vi "Layer Scan V4.vi"() -> ()   [LabVIEW 2024]
uses:
  <vilib>/DAQmx/write.llb/DAQmx Write (Analog 1D DBL NChan 1Samp).vi
  <vilib>/DAQmx/create/channels.llb/DAQmx Create Channel (AO-Voltage-Basic).vi
  <vilib>/DAQmx/miscellaneous.llb/DAQmx Fill In Error Info.vi
  <instrlib>/niScope/Configure/Trigger/niScope Configure Trigger Software.vi
  <instrlib>/niScope/Acquire/Fetch/niScope Fetch Cluster.vi
panel:
  in  "Channel Name 2":string="0" caption="Channel(s)"
  in  "Resource Name 2":refnum<k15>="Dev1" caption="Resource Name(s)"
  in  "Min. Sample Rate 2":dbl=10000000.0 caption="Min. Sample Rate" format="%#_6p"
  in  "Vertical Range (V) 2":dbl=2.0 caption="Vertical Range (V)" format="%_3g"
  out "Waveform from Scope":T1(graph)
  in  "Max. Points per Fetch":i32=1000
  in  "Plot Data?":bool=TRUE
  out "Last Points Fetched":i32
  out "Total Points Fetched":i32
  in  "Simulate?":bool
  out "decimated array 2":dbl[](array[numeric])
  out "decimated array":dbl[](array[numeric])
  out "Y coord filename":i32
  out "x coord file name":i32
  out "Filename Out":path
  in  "Data File Name":path
  in  "Data folder Path":path
  in  "X offset":dbl
  in  "Y offset":dbl
  in  "distance":dbl
  in  "Y Count":dbl
  in  "X Count":dbl
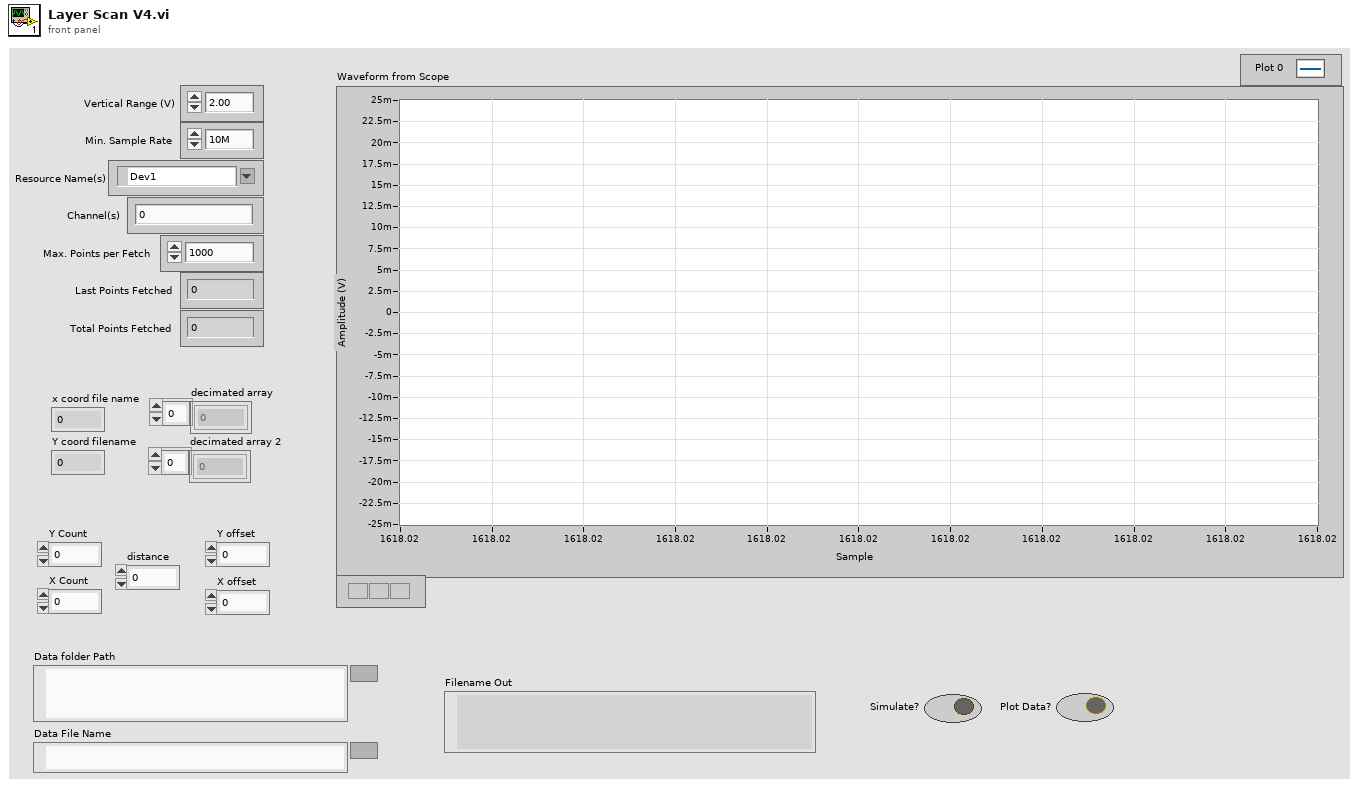
[diagram p1: front panel]
types:
  T1 = cluster{"relativeInitialX":dbl, "xIncrement":dbl, "wfm":dbl[]}
  T2 = cluster{"actualSamples":i32, "absoluteInitialX":dbl, "relativeInitialX":dbl, "xIncrement":dbl, "offset":dbl, "gain":dbl, "reserved1":dbl, "reserved2":dbl}
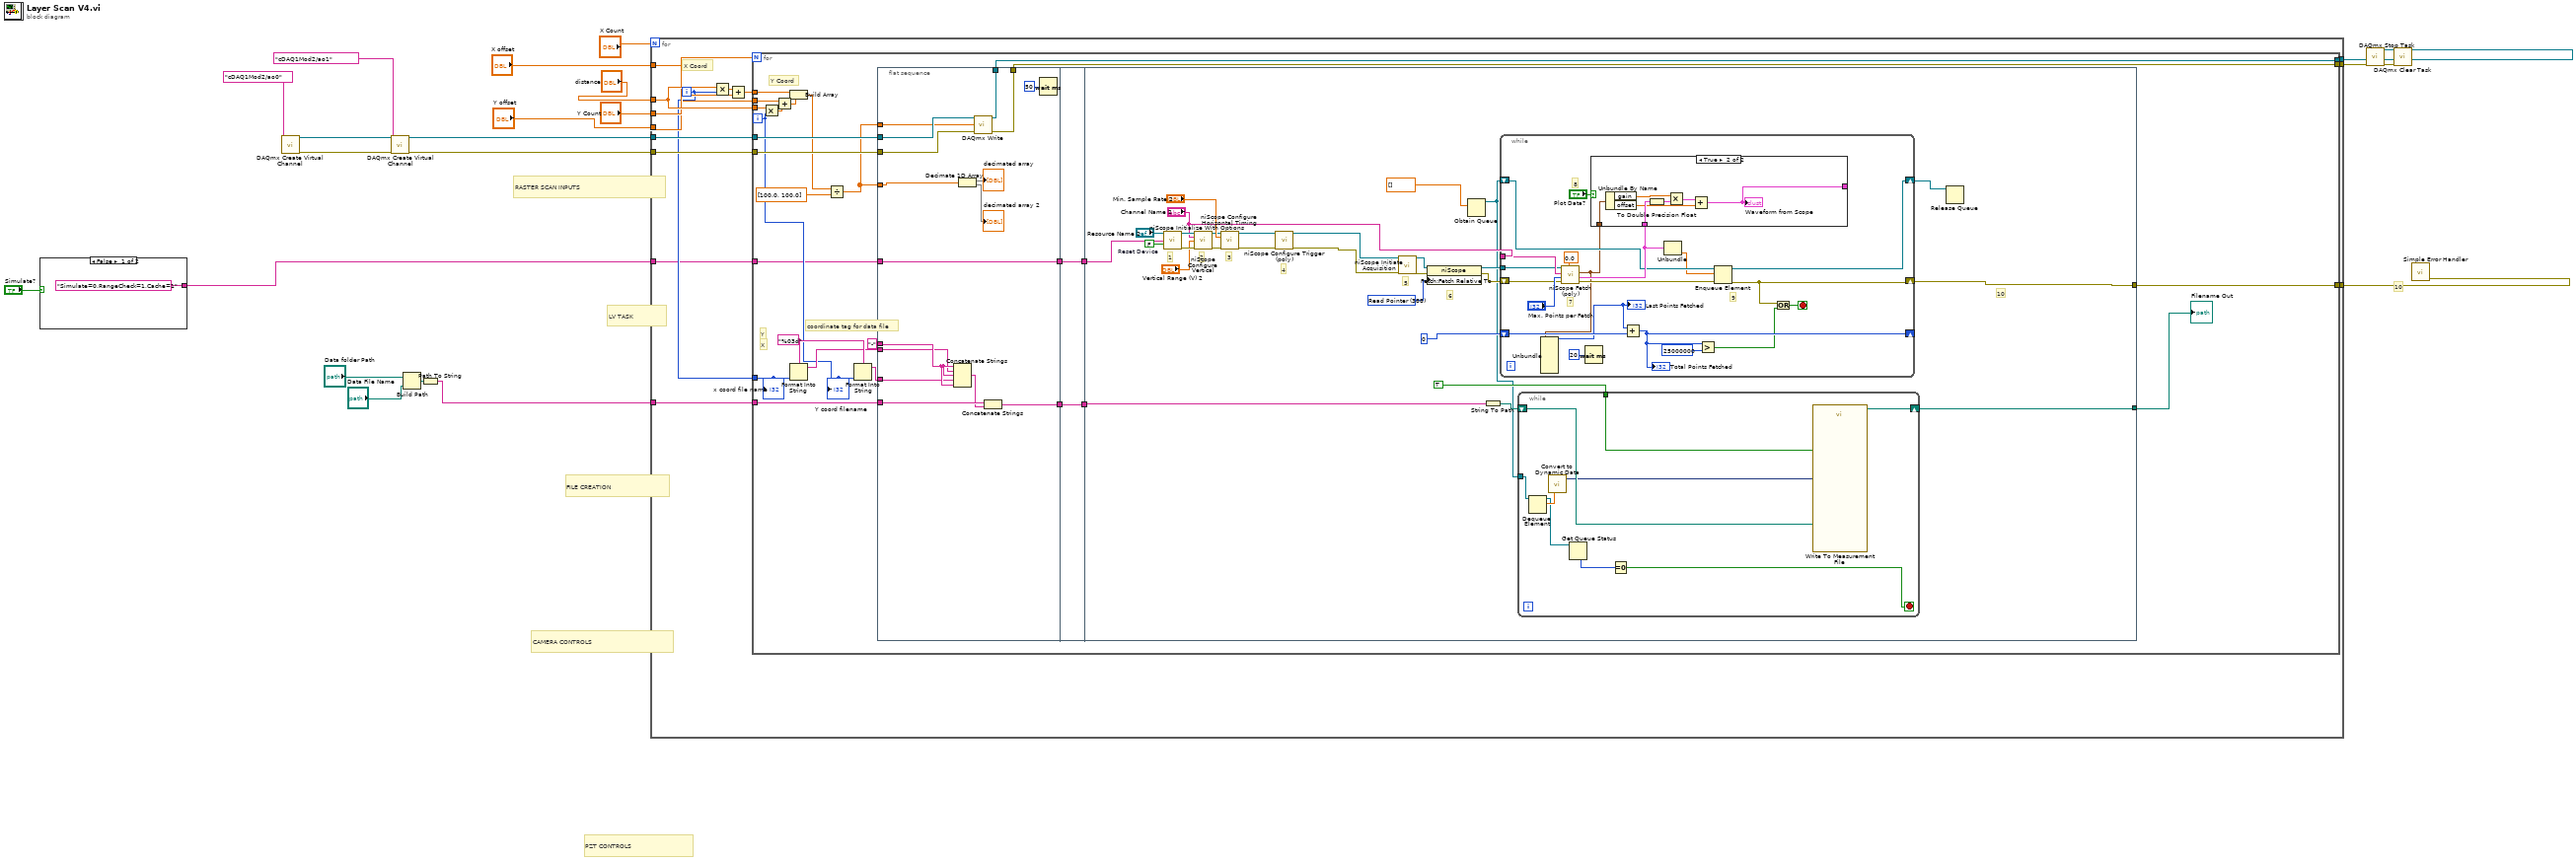
[diagram p0: block diagram]
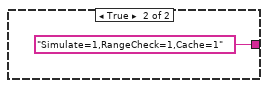
[diagram p2: hidden frame]
diagram:
  # "10"
  # "FILE CREATION"
  # "PZT CONTROLS"
  # "CAMERA CONTROLS"
  # "LV TASK"
  # "RASTER SCAN INPUTS"
  n1 = case shown="False" "Simulate?" {
    tunnel: ["Simulate=0,RangeCheck=1,Cache=1" ("option string") "Simulate=1,RangeCheck=1,Cache=1" ("option string")] -> w1
    frame False {
    }
    frame True {
    }
  }
  n2 = call-poly <vilib>:"DAQmx Create Virtual Channel.vi"("physical channels"=tag "cDAQ1Mod2/ao0") -> ("task out"=w15:refnum<k21>, "error out"=w14:errorcluster)  [unwired: 13 in]
  n3 = call-poly <vilib>:"DAQmx Create Virtual Channel.vi"("task in"=w15, "physical channels"=tag "cDAQ1Mod2/ao1", "error in"=w14) -> ("task out"=w13:refnum<k21>, "error out"=w12:errorcluster)  [unwired: 11 in]
  n4 = Build Path(base path="Data folder Path", name or relative path="Data File Name") -> (appended path=w5:path)
  n5 = Path To String(path=w5) -> (string=w4:string)
  n6 = for {
    N: "X Count" -> [_]
    tunnel: "distance" -> [w38]
    tunnel: "Y Count" -> [w37]
    tunnel: "Y offset" -> [w36]
    tunnel: "X offset" -> [w34]
    tunnel: w13 -> [w32]
    tunnel: w12 -> [w31]
    tunnel: [w30] -> w11
    tunnel: [w29] -> w10
    tunnel: [w28] -> w2
    tunnel: w4 -> [w27]
    tunnel: w1 -> [w25]
    i -> [w26]
    # "X Coord"
    n7 = Multiply(x=w38, y=w26) -> (x*y=w35:dbl)
    n8 = Add(x=w35, y=w34) -> (x+y=w33:dbl)
    n9 = for {
      N: w37 -> [_]
      tunnel: w38 -> [w64]
      tunnel: w36 -> [w62]
      tunnel: w33 -> [w61]
      tunnel: w32 -> [w59]
      tunnel: w31 -> [w58]
      tunnel: [w56] -> w30
      tunnel: [w55] -> w29
      tunnel: [w43] -> w28
      tunnel: w27 -> [w50]
      tunnel: w26 -> [w46]
      tunnel: w25 -> [w39]
      i -> [w45]
      w54 = "%03d" ("format string")
      # "coordinate tag for data file"
      # "X"
      # "Y"
      # "Y Coord"
      n10 = Multiply(x=w64, y=w45) -> (x*y=w63:dbl)
      n11 = Add(x=w62, y=w63) -> (x+y=w60:dbl)
      n12 = Format Into String(format string=w54, w46) -> (resulting string=w52:string)  [unwired: 2 in, 1 out]
      n13 = Build Array(w61, w60) -> (w57:dbl[])
      n14 = Divide(x=w57, y=dbl[] [100.0, 100.0]) -> (x/y=w44:dbl[])
      n15 = Format Into String(format string=w54, w45) -> (resulting string=w51:string)  [unwired: 2 in, 1 out]
      n16 = flat-sequence {
        tunnel: w59 -> [w79]
        tunnel: w58 -> [w78]
        tunnel: [w77] -> w56
        tunnel: [w76] -> w55
        tunnel: "-" ("string") -> [w75]
        tunnel: w52 -> [w74]
        tunnel: w51 -> [w73]
        tunnel: w50 -> [w72]
        tunnel: [w70] -> w49
        tunnel: w44 -> [w69]
        tunnel: w44 -> [w68]
        tunnel: [w65] -> w41
        tunnel: w39 -> [w65]
        tunnel: w49 -> [w82]
        tunnel: [w82] -> w48
        tunnel: w41 -> [w81]
        tunnel: [w81] -> w40
        tunnel: w48 -> [w110]
        tunnel: [w83] -> w43
        tunnel: [w87] -> w42
        tunnel: w40 -> [w90]
        frame #0 {
          n17 = Concatenate Strings(w75, w74, w75, w73, w75) -> (w71:string)
          n18 = Decimate 1D Array(w68) -> (→"decimated array":dbl[], →"decimated array 2":dbl[])
          n19 = call-poly <vilib>:"DAQmx Write.vi"("task/channels in"=w79, "data"=w69, "error in"=w78) -> ("task out"=w77:refnum<k21>, "error out"=w76:errorcluster)  [unwired: 10 in, 1 out]
          n20 = Concatenate Strings(w72, w71) -> (w70:string)
          n21 = Wait (ms)(milliseconds to wait=u32 50) -> ()  [unwired: 1 out]
        }
        frame #1 {
        }
        frame #2 {
          w101 = FALSE  # Reset Device
          w106 = 388 items=["Start"=482, "Trigger"=483, "Pretrigger"=477, "Now"=481, "Read Pointer"=388] ("Fetch:Fetch Relative To")
          # "4"
          # "3"
          # "2"
          # "1"
          # "10"
          # "6"
          # "5"
          n22 = call <instrlib>:"niScope Initialize With Options.vi"("resource name"="Resource Name 2", "option string"=w90, "reset device"=w101) -> ("instrument handle"=w103:refnum<k15>, "error out"=w102:errorcluster)  [unwired: 11 in]
          n23 = call <instrlib>:"niScope Configure Vertical.vi"("instrument handle"=w103, "channels"="Channel Name 2", "vertical range"="Vertical Range (V) 2", "error in"=w102) -> ("instrument handle out"=w95:refnum<k15>, "error out"=w94:errorcluster)  [unwired: 10 in]
          n24 = call <instrlib>:"niScope Configure Horizontal Timing.vi"("instrument handle"=w95, "min sample rate"="Min. Sample Rate 2", "error in"=w94) -> ("instrument handle out"=w99:refnum<k15>, "error out"=w100:errorcluster)  [unwired: 11 in]
          n25 = call-poly <instrlib>:"niScope Configure Trigger (poly).vi"("instrument handle"=w99, "error in"=w100) -> ("instrument handle out"=w92:refnum<k15>, "error out"=w91:errorcluster)  [unwired: 12 in]
          n26 = call <instrlib>:"niScope Initiate Acquisition.vi"("instrument handle"=w92, "error in"=w91) -> ("instrument handle out"=w107:refnum<k15>, "error out"=w108:errorcluster)  [unwired: 12 in]
          n27 = property class="niScope"(reference=w107, error in=w108, "Fetch:Fetch Relative To"=w106) -> (reference out=w104:refnum<k15>, error out=w105:errorcluster)
          n28 = Obtain Queue(element data type=dbl[] []) -> (queue out=w85:refnum<queue>)  [unwired: 4 in, 2 out]
          n29 = String To Path(string=w110) -> (path=w88:path)
          n30 = while {
            shift-left: 0 -> [w139]
            shift-right: [w130] -> _
            tunnel: "Channel Name 2" -> [w137]
            tunnel: w104 -> [w133]
            shift-right: [w126] -> w83
            shift-left: w105 -> [w132]
            shift-right: [w122] -> w86
            shift-left: w85 -> [w124]
            stop <- w138 stop-if-true
            # "9"
            # "8"
            # "7"
            n31 = call-poly <instrlib>:"niScope Fetch (poly).vi"("timeout"=0.0, "error in"=w132, "numSamples"="Max. Points per Fetch", "channels"=w137, "instrument handle"=w133) -> ("error out"=w127:errorcluster, "waveform"=w125:T1, "wfm info"=w121:T2)  [unwired: 3 in, 1 out]
            n32 = Unbundle(w121) -> ("actualSamples"=w120:i32)  [unwired: 7 out]
            "Last Points Fetched" <- w120
            n33 = Wait (ms)(milliseconds to wait=u32 20) -> ()  [unwired: 1 out]
            n34 = case shown="True" "Plot Data?" {
              tunnel: w125 -> [_ w145]
              tunnel: w121 -> [_ w146]
              tunnel: [_ w140] -> _
              frame False {
              }
              frame True {
                n35 = Unbundle By Name(w146) -> ("gain"=w144:dbl, "offset"=w142:dbl)
                n36 = To Double Precision Float(number=w145) -> (double precision float=w141:T1)
                n37 = Multiply(x=w144, y=w141) -> (x*y=w143:T1)
                n38 = Add(x=w143, y=w142) -> (x+y=w140:T1)
                "Waveform from Scope" <- w140
              }
            }
            n39 = Add(x=w120, y=w139) -> (x+y=w130:i32)
            "Total Points Fetched" <- w130
            n40 = Unbundle(w125) -> ("wfm"=w123:dbl[])  [unwired: 2 out]
            n41 = Greater?(x=w130, y=25000000) -> (0:w128:bool)
            n42 = Enqueue Element(queue=w124, element=w123, error in (no error)=w127) -> (queue out=w122:refnum<queue>, error out=w126:errorcluster)  [unwired: 1 in, 1 out]
            n43 = Or(x=w126, y=w128) -> (x .or. y?=w138:bool)
          }
          n44 = while {
            tunnel: TRUE ("Enable") -> [w119]
            tunnel: w85 -> [w115]
            shift-right: [w117] -> w87
            shift-left: w88 -> [w118]
            stop <- w111 stop-if-true
            n45 = Dequeue Element(queue=w115) -> (queue out=w113:refnum<queue>, element=w116:dbl[])  [unwired: 2 in, 2 out]
            n46 = call "Convert to Dynamic Data"("Array"=w116) -> ("Dynamic Data Type"=w114:dynamicdata)  [unwired: 3 in]
            n47 = Get Queue Status(queue=w113) -> (# elements in queue=w112:i32)  [unwired: 2 in, 7 out]
            n48 = Equal To 0?(x=w112) -> (x = 0?=w111:bool)
            n49 = call "Write To Measurement File"("Signals"=w114, "Enable"=w119, "Filename"=w118) -> ("Filename Out"=w117:path)  [unwired: 14 in, 2 out]
          }
          n50 = Release Queue(queue=w86) -> ()  [unwired: 2 in, 3 out]
        }
      }
      "Filename Out" <- w42
      "x coord file name" <- w46
      "Y coord filename" <- w45
    }
  }
  n51 = call <vilib>:"DAQmx Stop Task.vi"("task/channels in"=w11, "error in"=w10) -> ("task out"=w9:refnum<k21>, "error out"=w8:errorcluster)  [unwired: 12 in]
  n52 = call <vilib>:"DAQmx Clear Task.vi"("task in"=w9, "error in"=w8) -> ()  [unwired: 13 in, 1 out]
  n53 = call <vilib>:"Simple Error Handler.vi"("error in (no error)"=w2) -> ()  [unwired: 4 in, 5 out]
